vi "Many Current Ramp Com.vi"() -> (0 "Command text":string[][](array[string]))   [LabVIEW 2021]
uses:
  CurrentRamp Instrument.ctl
  CurrentRamp.ctl
panel:
  in  "interval(sec)":dbl=0.5 min=0.1 step=0.1
  in  "wait after each sweep (sec)":i32
  in  "CurrentRamp":T1={"VISA Resource Name"="", "extra wait"=1, "start"=1e-12, "end"=0.002, "Sweep Time (H:M:S)"=1800.0, "Log Linear"=FALSE, "interval(sec)"=0.5, "Select Instrument"=enum."Keithley 6221 Coarse"} {"interval(sec)" min=0.5 step=0.1; "Sweep Time (H:M:S)" format="%<%H:%M:%S>t"; "extra wait" min=0; "start" format="%#.7e"; "end" format="%#.7e"}
  out "loop array":dbl[][](array[numeric])
  in  "next":bool
  in  "cancel":bool
  in  "Generate":bool
  in  "Number of Interval":dbl
  in  "Delta Current (A)":dbl
  in  "Sweep time":dbl=1.0 min=1.0 max=359999.0 format="%<%H:%M:%S>t"
  in  "Final Start Current (A)":dbl
  in  "Initial Start Current (A)":dbl
  in  "Select Instrument":T2
  in  "VISA Resource Name":refnum<visa-resource-name>
  in  "Log Linear":bool
  in  "Array":dbl[][](array[numeric]) format="%#_4e"
  # "Multiple Current Ramp Sequence Generator"
  # "Log"
  # "Linear"
  # "(Start Current + Delta Current = End Current)"
  # "seconds"
  # "Minimum update between two points of sweep:"
  # "generates multiple current ramp values for the sequence, see belolw.\nIf you like it click \"Good, use this!\". You can also modify the values directly from the following array."
  # "Start Current (A)"
  # "End Current (A)"
  # "Sweep time (sec)"
  # "Current Ramp"
  # "Instrument \nAddress"
  # "Select\nInstrument"
  # "Log"
  # "End Current (A)"
  # "Sweep Time (HH:MM:SS)"
  # "Start Current (A)"
  # "Linear"
  # "seconds"
  # "Minimum Time Interval Between Two Points"
  # "seconds"
  # "AND wait extra"
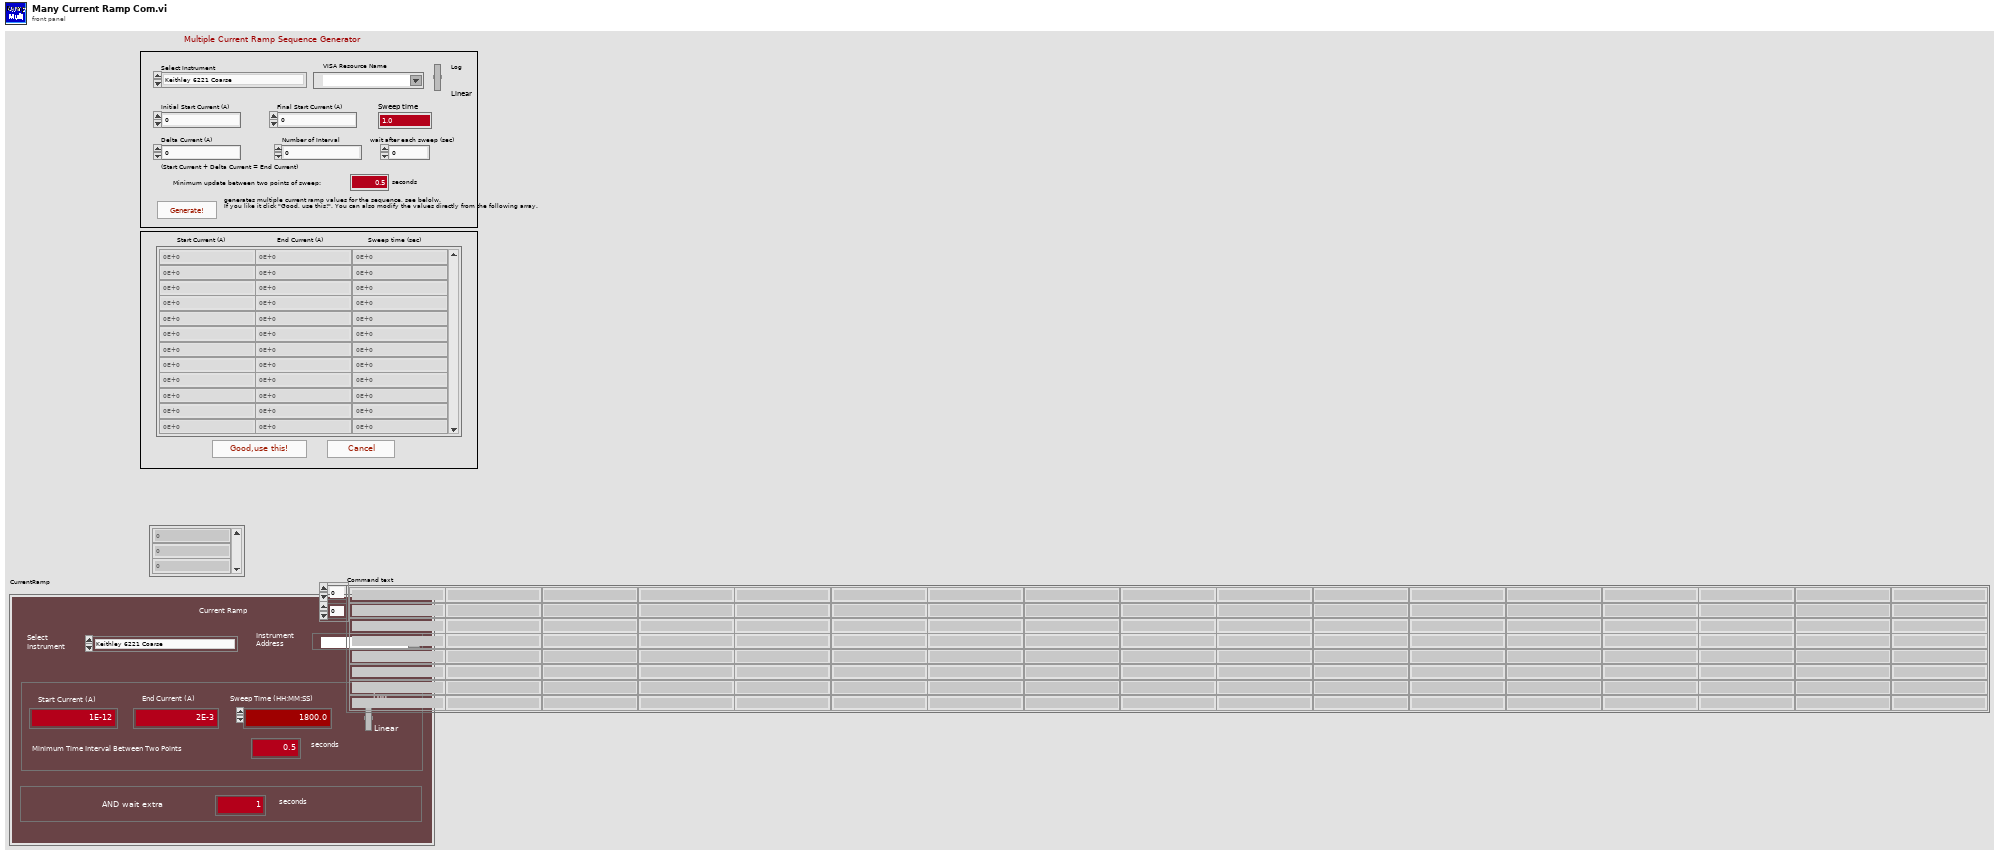
[diagram p1: front panel]
types:
  T1 = typedef "CurrentRamp.ctl" = cluster{"VISA Resource Name":refnum<visa-resource-name>, "extra wait":i32, "start":dbl, "end":dbl, "Sweep Time (H:M:S)":dbl, "Log Linear":bool, "interval(sec)":dbl, "Select Instrument":T2}
  T2 = typedef "CurrentRamp Instrument.ctl" = enum16{"Keithley 6221 Coarse"}
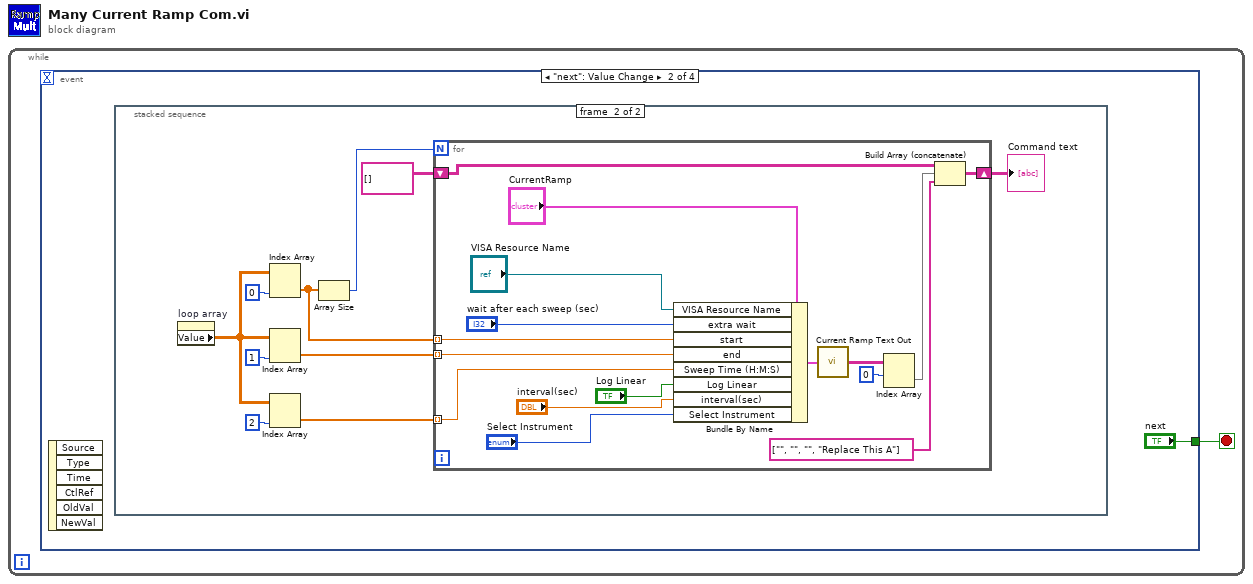
[diagram p0: block diagram]
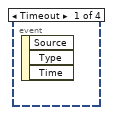
[diagram p2: hidden frame]
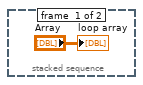
[diagram p3: hidden frame]
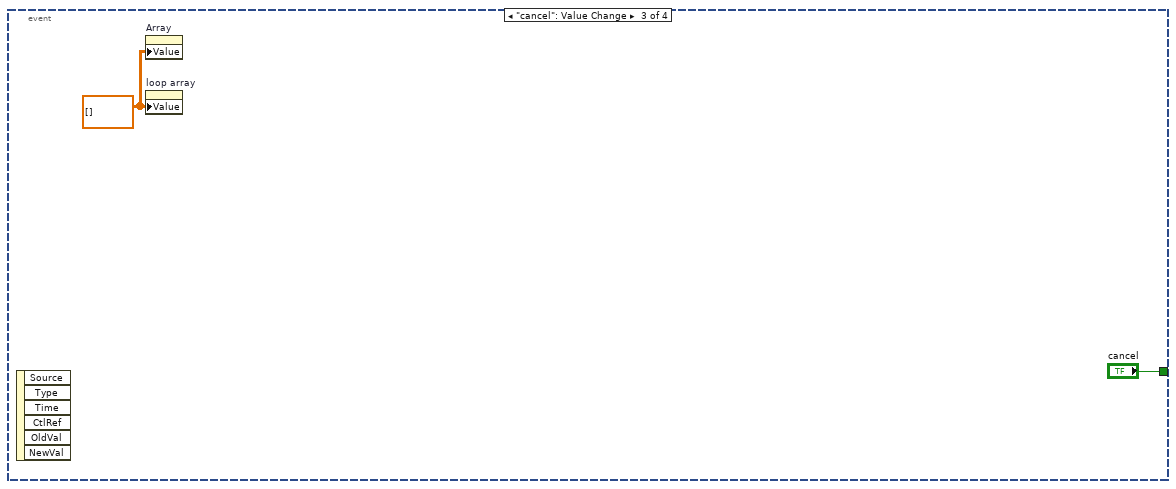
[diagram p4: hidden frame]
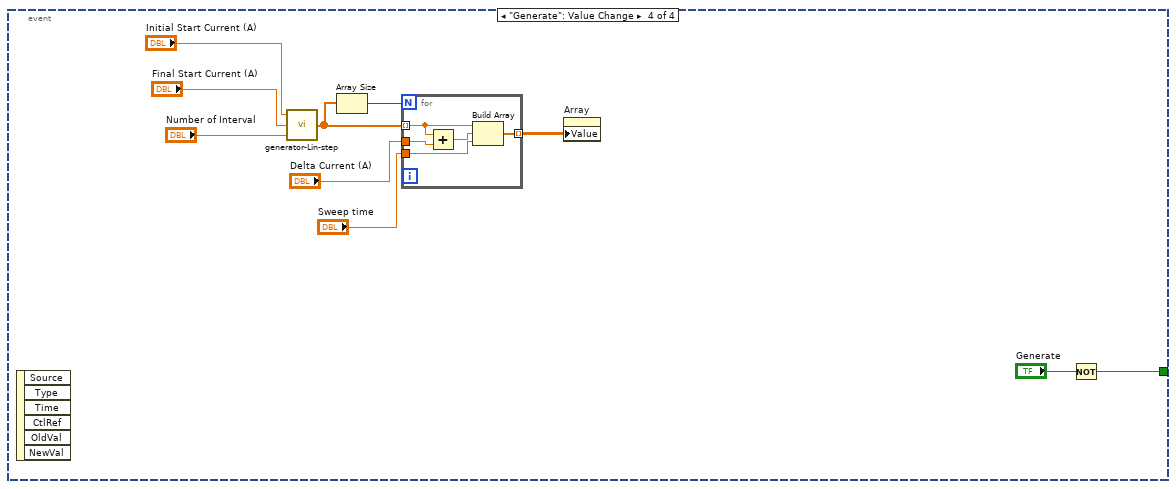
[diagram p5: hidden frame]
diagram:
  n1 = while {
    stop <- w1 stop-if-true
    n2 = event shown="[1] \"next\": Value Change" {
      selector: _ -> [_ _ _ _]
      dyn-events: _ -> [_ _ _ _]
      timeout: _ -> [_ _ _ _]
      tunnel: [_ "next" "cancel" w36] -> w1
      event Timeout {
        n3 = event-data() -> ()  [unwired: 1 in, 3 out]
      }
      event "next": Value Change {
        n4 = event-data() -> ()  [unwired: 1 in, 6 out]
        n5 = stacked-sequence {
          frame #0 {
            "loop array" <- "Array"
          }
          frame #1 {
            n6 = property on="loop array" class="Arr (strict)"() -> ("Value"=w10:dbl[][])  [unwired: 2 in, 2 out]
            n7 = Index Array(array=w10, index (col)=0 ("disabled index (col)")) -> (element=w9:dbl[])  [unwired: 1 in]
            n8 = Index Array(array=w10, index (col)=1 ("disabled index (col)")) -> (element=w8:dbl[])  [unwired: 1 in]
            n9 = Index Array(array=w10, index (col)=2 ("disabled index (col)")) -> (element=w7:dbl[])  [unwired: 1 in]
            n10 = Array Size(array=w9) -> (size(s)=w6:i32)
            n11 = for {
              N: w6 -> [_]
              tunnel: w9 -> [w25] mode=indexing
              tunnel: w8 -> [w24] mode=indexing
              tunnel: w7 -> [w23] mode=indexing
              shift-right: [w15] -> w5
              shift-left: string[][] [] -> [w14]
              n12 = Bundle By Name(cluster="CurrentRamp", "VISA Resource Name"="VISA Resource Name", "extra wait"="wait after each sweep (sec)", "start"=w25, "end"=w24, "Sweep Time (H:M:S)"=w23, "Log Linear"="Log Linear", "interval(sec)"="interval(sec)", "Select Instrument"="Select Instrument") -> (w28:T1)
              n13 = call "Current Ramp Text Out.vi"("CurrentRamp"=w28) -> ("Command text"=w19:string[][])
              n14 = Index Array(array=w19, index (row)=0) -> (element=w17:string[])  [unwired: 1 in]
              n15 = Build Array (concatenate)(w14, w17, string[] ["", "", "", "Replace This A"]) -> (w15:string[][])
            }
            "Command text" <- w5
          }
        }
      }
      event "cancel": Value Change {
        w30 = dbl[][] [] ("Array")
        n16 = event-data() -> ()  [unwired: 1 in, 6 out]
        n17 = property on="Array" class="Arr (strict)"("Value"=w30) -> ()  [unwired: 2 in, 2 out]
        n18 = property on="loop array" class="Arr (strict)"("Value"=w30) -> ()  [unwired: 2 in, 2 out]
      }
      event "Generate": Value Change {
        n19 = event-data() -> ()  [unwired: 1 in, 6 out]
        n20 = call "generator-Lin-step.vi"("step"="Number of Interval", "end"="Final Start Current (A)", "start"="Initial Start Current (A)") -> ("Array"=w33:dbl[])
        n21 = Array Size(array=w33) -> (size(s)=w37:i32)
        n22 = for {
          N: w37 -> [_]
          tunnel: w33 -> [w46] mode=indexing
          tunnel: "Delta Current (A)" -> [w45]
          tunnel: "Sweep time" -> [w43]
          tunnel: [w42] -> w32 mode=indexing
          n23 = Add(x=w46, y=w45) -> (x+y=w44:dbl)
          n24 = Build Array(w46, w44, w43) -> (w42:dbl[])
        }
        n25 = property on="Array" class="Arr (strict)"("Value"=w32) -> ()  [unwired: 2 in, 2 out]
        n26 = Not(x="Generate") -> (.not. x?=w36:bool)
      }
    }
  }
